vi "mod_createSeeds.vi"(3 "Reset? (T)":bool=TRUE, 4 "# of seeds to create":i32=1, 5 "Allow Neg if not already? (T)":bool=TRUE, 6 "seed in (0xFFFFFFFF)":i32=-1 format="%.0x") -> (0 "Next seed":i32 format="%.0x", 1 "First Seed":i32 format="%.0x", 2 "Seeds":i32[](array[numeric]) format="%.0x")   [LabVIEW 2020, in "niDMT.lvlib"]
uses:
  <vilib>/addons/Modulation/niDMT.lvlib
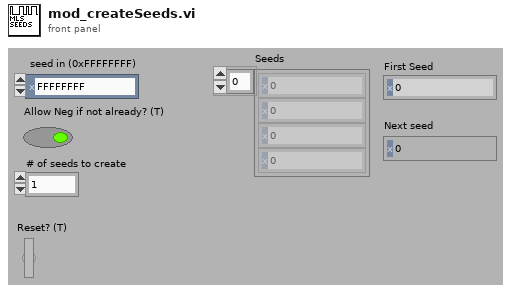
[diagram p1: front panel]
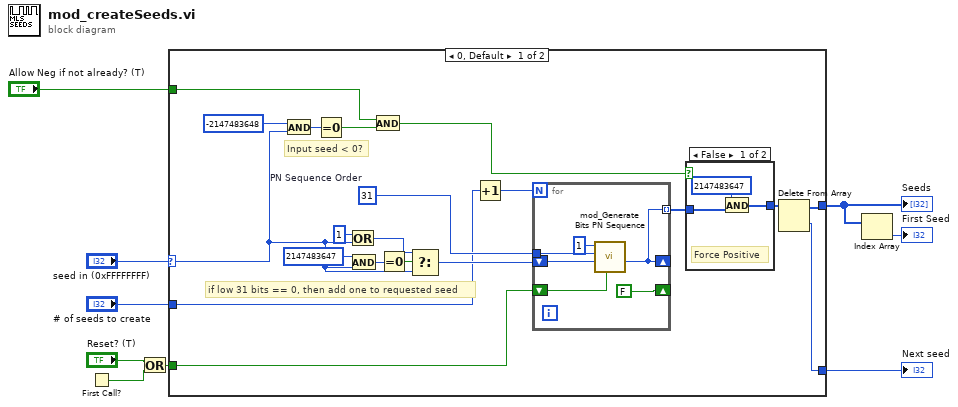
[diagram p0: block diagram]
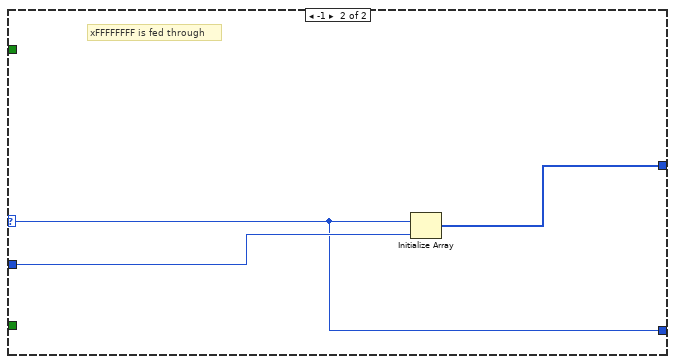
[diagram p3: hidden frame]
diagram:
  n1 = First Call?() -> (First Call?: T/F=w3:bool)
  n2 = Or(x="Reset? (T)", y=w3) -> (x .or. y?=w2:bool)
  n3 = case shown="0, Default" "seed in (0xFFFFFFFF)" {
    selector: "seed in (0xFFFFFFFF)" -> [w20 w41]
    tunnel: [w10 w41] -> w8
    tunnel: "# of seeds to create" -> [w15 w42]
    tunnel: [w11 w40] -> w6
    tunnel: w2 -> [w16 _]
    tunnel: "Allow Neg if not already? (T)" -> [w17 _]
    frame 0, Default {
      w25 = 31  # PN Sequence Order
      # "if low 31 bits == 0, then add one to requested seed"
      # "Input seed < 0?"
      n4 = And(x=-2147483648, y=w20) -> (x .and. y?=w28:i32)
      n5 = Equal To 0?(x=w28) -> (x = 0?=w27:bool)
      n6 = Or(x=1 ("t"), y=w20) -> (x .or. y?=w21:i32)
      n7 = And(x=2147483647, y=w20) -> (x .and. y?=w24:i32)
      n8 = And(x=w17, y=w27) -> (x .and. y?=w26:bool)
      n9 = Equal To 0?(x=w24) -> (x = 0?=w23:bool)
      n10 = Select(t=w21, s=w23, f=w20) -> (s? t:f=w19:i32)
      n11 = Increment(x=w15) -> (x+1=w14:i32)
      n12 = for {
        N: w14 -> [_]
        tunnel: w25 -> [w35]
        shift-right: [w33] -> _
        shift-left: w19 -> [w34]
        tunnel: [w33] -> w13 mode=indexing
        shift-right: [FALSE] -> _
        shift-left: w16 -> [w31]
        n13 = call <vilib>:"mod_Generate Bits PN Sequence.vi"("Reset? (T)"=w31, "seed in (0xD6BF7DF2)"=w34, "PN Sequence Order (9)"=w35, "Total Bits"=1) -> ("seed out"=w33:u32)  [unwired: 7 out]
      }
      n14 = case shown="False" w26 {
        tunnel: [w37 w39] -> w12
        tunnel: w13 -> [w36 w39]
        frame False {
          # "Force Positive"
          n15 = And(x=u32 2147483647, y=w36) -> (x .and. y?=w37:u32[])
        }
        frame True {
        }
      }
      n16 = Delete From Array(array=w12) -> (deleted portion=w10:u32, array with subset deleted=w11:u32[])  [unwired: 2 in]
    }
    frame -1 {
      # "xFFFFFFFF is fed through"
      n17 = Initialize Array(w41, w42) -> (w40:i32[])
    }
  }
  "Next seed" <- w8
  "Seeds" <- w6
  n18 = Index Array(array=w6) -> (element=→"First Seed":u32)  [unwired: 1 in]
